vi "ECOG-Initialize.vi"(0 "params":T1) -> (4 "task out":refnum<k21>, 8 "nread":i32, 15 "error out":errorcluster)   [LabVIEW 2020]
uses:
  Typedefs/ECOG-Parameters.ctl
  <vilib>/DAQmx/create/channels.llb/DAQmx Create Channel (AI-Voltage-Basic).vi
  <vilib>/DAQmx/configure/timing.llb/DAQmx Timing (Sample Clock).vi
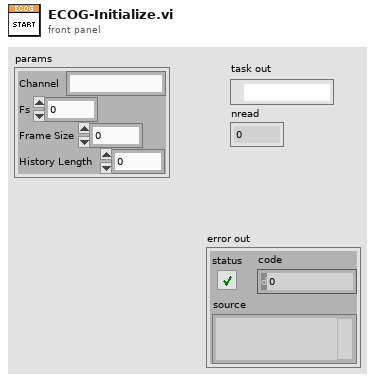
[diagram p1: front panel]
types:
  T1 = typedef "ECOG-Parameters.ctl" = cluster{"Channel":string, "Fs":dbl, "Frame Size":dbl, "History Length":dbl}
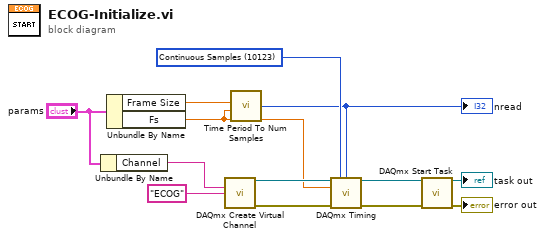
[diagram p0: block diagram]
diagram:
  w8 = 10123 items=["Finite Samples"=10178, "Continuous Samples"=10123, "Hardware Timed Single Point"=12522] ("sample mode")
  n1 = Unbundle By Name("params") -> ("Channel"=w13:string)
  n2 = Unbundle By Name("params") -> ("Frame Size"=w7:dbl, "Fs"=w6:dbl)
  n3 = call-poly <vilib>:"DAQmx Create Virtual Channel.vi"("physical channels"=w13, "name to assign"="ECOG") -> ("task out"=w11:refnum<k21>, "error out"=w10:errorcluster)  [unwired: 12 in]
  n4 = call "Time Period To Num Samples.vi"("Duration (ms)"=w7, "Sampling rate (Hz)"=w6) -> ("Samples"=w5:i32)  [unwired: 5 in]
  "nread" <- w5
  n5 = call-poly <vilib>:"DAQmx Timing.vi"("task/channels in"=w11, "sample mode"=w8, "samples per channel"=w5, "rate"=w6, "error in"=w10) -> ("task out"=w4:refnum<k21>, "error out"=w3:errorcluster)  [unwired: 9 in]
  n6 = call <vilib>:"DAQmx Start Task.vi"("task/channels in"=w4, "error in"=w3) -> ("task out"=→"task out":refnum<k21>, "error out"=→"error out":errorcluster)  [unwired: 12 in]
